vi "ETAS_Driver.vi"(7 "IP Address":string, 8 "Loop In":u32, 9 "error In":errorcluster, 10 "Con ID In":refnum<k24>, 11 "Connect":bool) -> (0 "Loop Out":u32, 1 "error out":errorcluster, 2 "Con ID Out":refnum<k24>, 3 "ETAS Out":dbl[](array[numeric]))   [LabVIEW 2014]
uses:
  C:/Users/JonnyS/Desktop/OMEGA_14/Drivers/ETASdigital.dll
  ETASdigital.dll
panel:
  # "ETAS Driver Vi"
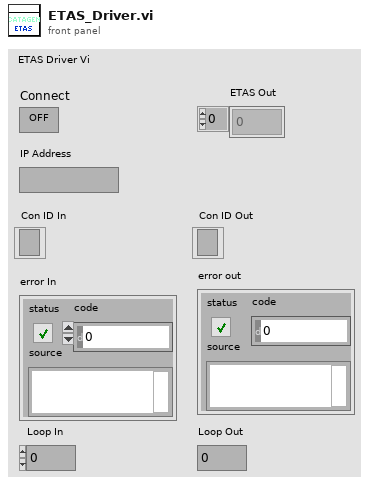
[diagram p1: front panel]
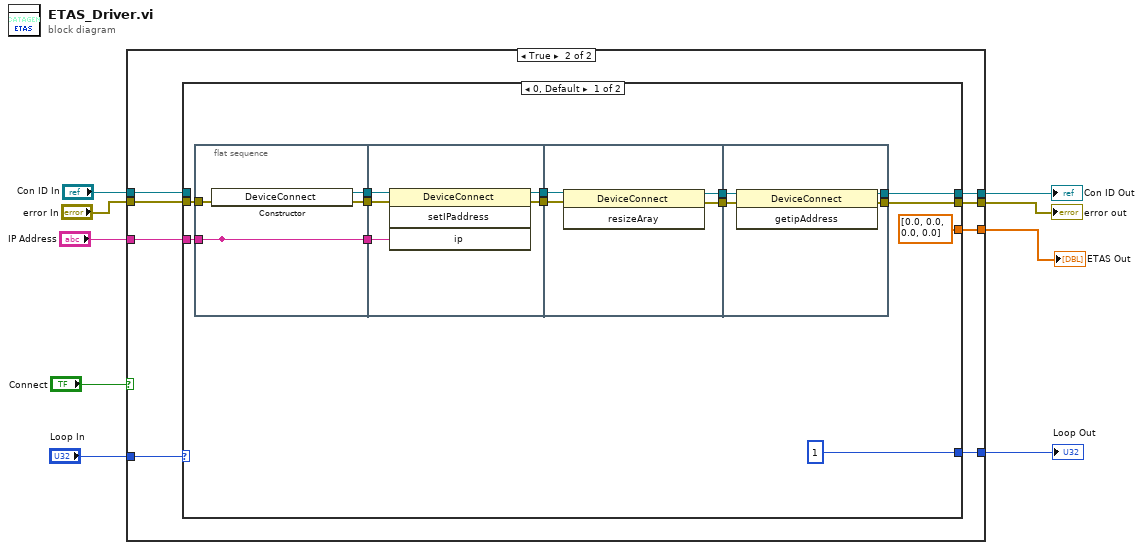
[diagram p0: block diagram]
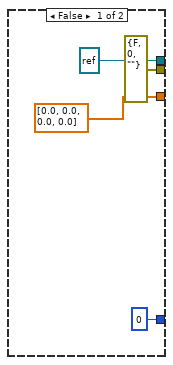
[diagram p2: hidden frame]
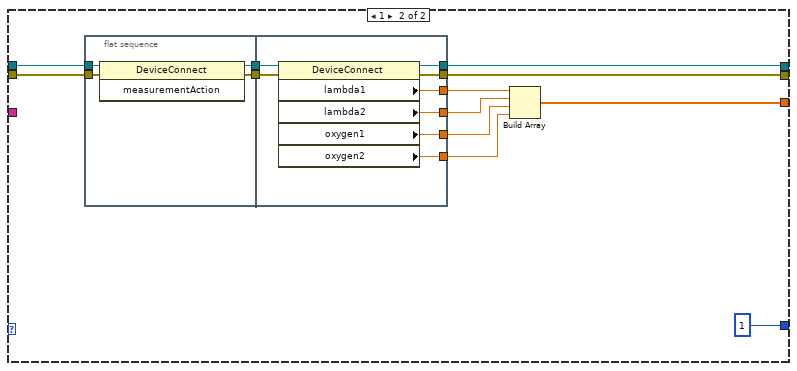
[diagram p3: hidden frame]
diagram:
  n1 = case shown="True" "Connect" {
    tunnel: [u32 0 ("number") w21] -> w3
    tunnel: [refnum<k24> refnum ("new reference") w20] -> w8
    tunnel: [errorcluster {"status"=FALSE, "code"=0, "source"=""} ("error out") w19] -> w7
    tunnel: "error In" -> [_ w18]
    tunnel: "Con ID In" -> [_ w17]
    tunnel: [dbl[] [0.0, 0.0, 0.0, 0.0] w16] -> w4
    tunnel: "Loop In" -> [_ w15]
    tunnel: "IP Address" -> [_ w14]
    frame False {
    }
    frame True {
      n2 = case shown="0, Default" w15 {
        tunnel: [u32 1 ("number") u32 1 ("number")] -> w21
        tunnel: [w28 w53] -> w20
        tunnel: [w27 w52] -> w19
        tunnel: w18 -> [w26 w62]
        tunnel: w17 -> [_ w61]
        tunnel: [dbl[] [0.0, 0.0, 0.0, 0.0] w54] -> w16
        tunnel: w14 -> [w22 _]
        frame 0, Default {
          n3 = flat-sequence {
            tunnel: [w38] -> w32
            tunnel: [w37] -> w31
            tunnel: w26 -> [w36]
            tunnel: [w35] -> _
            tunnel: [w35] -> w23
            tunnel: w22 -> [w35]
            tunnel: [w41] -> w33
            tunnel: w32 -> [w43]
            tunnel: w31 -> [w42]
            tunnel: [w40] -> w24
            tunnel: w23 -> [w39]
            tunnel: w33 -> [w47]
            tunnel: [w45] -> w30
            tunnel: [w44] -> w29
            tunnel: w24 -> [w46]
            tunnel: w30 -> [w51]
            tunnel: w29 -> [w50]
            tunnel: [w49] -> w28
            tunnel: [w48] -> w27
            frame #0 {
              n4 = constructor class="DeviceConnect"(error in=w36) -> (reference out=w38:refnum<k24>, error out=w37:errorcluster)  [unwired: 2 in, 1 out]
            }
            frame #1 {
              n5 = invoke class="DeviceConnect" method="setIPaddress"(reference=w43, error in=w42, "ip"=w39) -> (reference out=w41:refnum<k24>, error out=w40:errorcluster)  [unwired: 1 in, 2 out]
            }
            frame #2 {
              n6 = invoke class="DeviceConnect" method="resizeAray"(reference=w47, error in=w46) -> (reference out=w45:refnum<k24>, error out=w44:errorcluster)  [unwired: 1 in, 1 out]
            }
            frame #3 {
              n7 = invoke class="DeviceConnect" method="getipAddress"(reference=w51, error in=w50) -> (reference out=w49:refnum<k24>, error out=w48:errorcluster)  [unwired: 1 in, 1 out]
            }
          }
        }
        frame 1 {
          n8 = flat-sequence {
            tunnel: w62 -> [w67]
            tunnel: w61 -> [w66]
            tunnel: [w65] -> w60
            tunnel: [w64] -> w59
            tunnel: w60 -> [w74]
            tunnel: w59 -> [w75]
            tunnel: [w73] -> w58
            tunnel: [w72] -> w57
            tunnel: [w71] -> w56
            tunnel: [w70] -> w55
            tunnel: [w69] -> w53
            tunnel: [w68] -> w52
            frame #0 {
              n9 = invoke class="DeviceConnect" method="measurementAction"(reference=w66, error in=w67) -> (reference out=w64:refnum<k24>, error out=w65:errorcluster)  [unwired: 1 in, 1 out]
            }
            frame #1 {
              n10 = property class="DeviceConnect"(reference=w75, error in=w74) -> (reference out=w69:refnum<k24>, error out=w68:errorcluster, "lambda1"=w73:dbl, "lambda2"=w72:dbl, "oxygen1"=w71:dbl, "oxygen2"=w70:dbl)
            }
          }
          n11 = Build Array(w58, w57, w56, w55) -> (w54:dbl[])
        }
      }
    }
  }
  "Con ID Out" <- w8
  "error out" <- w7
  "ETAS Out" <- w4
  "Loop Out" <- w3
